vi "TLA_Assembling.vi"(5 "User":string, 6 "stnID":i32, 7 "ProcessIDList":string, 8 "error in (no error)":errorcluster caption="错误输入（无错误）", 9 "JobNo":string, 10 "PCBID":string, 11 "Traceability 引用句柄":refnum<k24>) -> (0 "error out":errorcluster caption="错误输出", 2 ".NET:System.Data.DataTable":T1 {"RemotingFormat" items=["Xml", "Binary"]}, 3 "Traceability 引用句柄输出":refnum<k24>)   [LabVIEW 2014, in "Traceability.lvlib"]
uses:
  D:/webservice/Traceability.dll
  Traceability.dll
  System.Data
  Traceability.lvlib
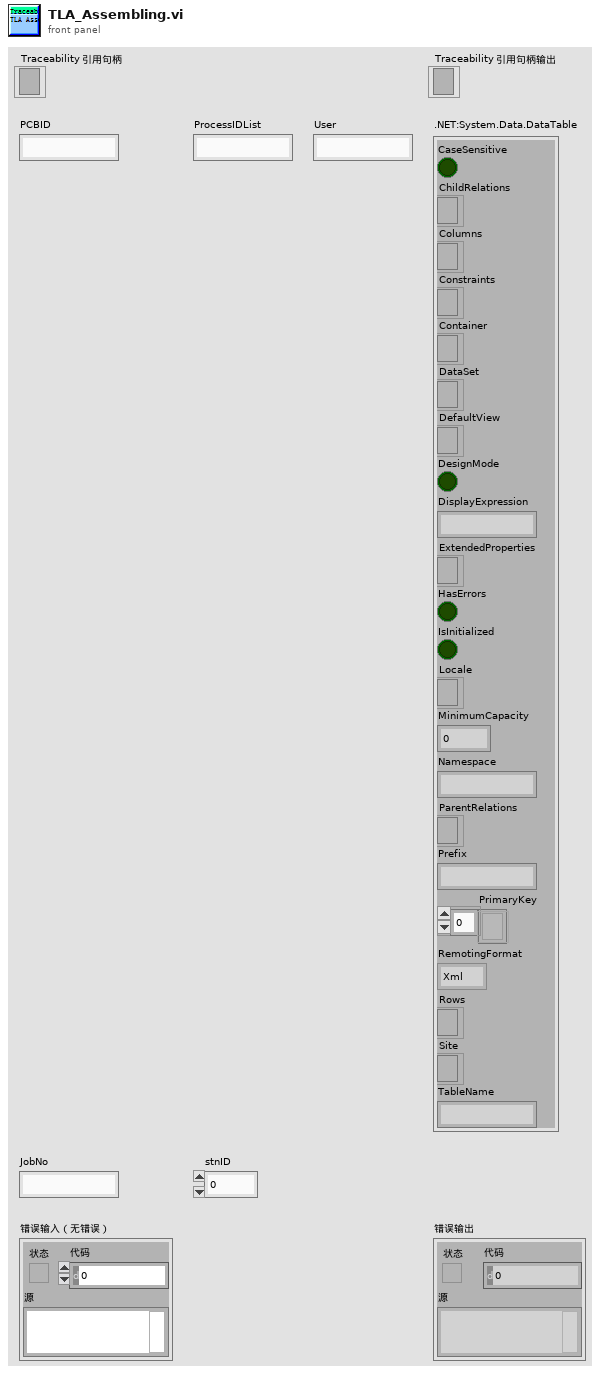
[diagram p1: front panel]
types:
  T1 = cluster{"CaseSensitive":bool, "ChildRelations":refnum<k24>, "Columns":refnum<k24>, "Constraints":refnum<k24>, "Container":refnum<k24>, "DataSet":refnum<k24>, "DefaultView":refnum<k24>, "DesignMode":bool, "DisplayExpression":string, "ExtendedProperties":refnum<k24>, "HasErrors":bool, "IsInitialized":bool, "Locale":refnum<k24>, "MinimumCapacity":i32, "Namespace":string, "ParentRelations":refnum<k24>, "Prefix":string, "PrimaryKey":refnum<k24>[], "RemotingFormat":i32, "Rows":refnum<k24>, "Site":refnum<k24>, "TableName":string}
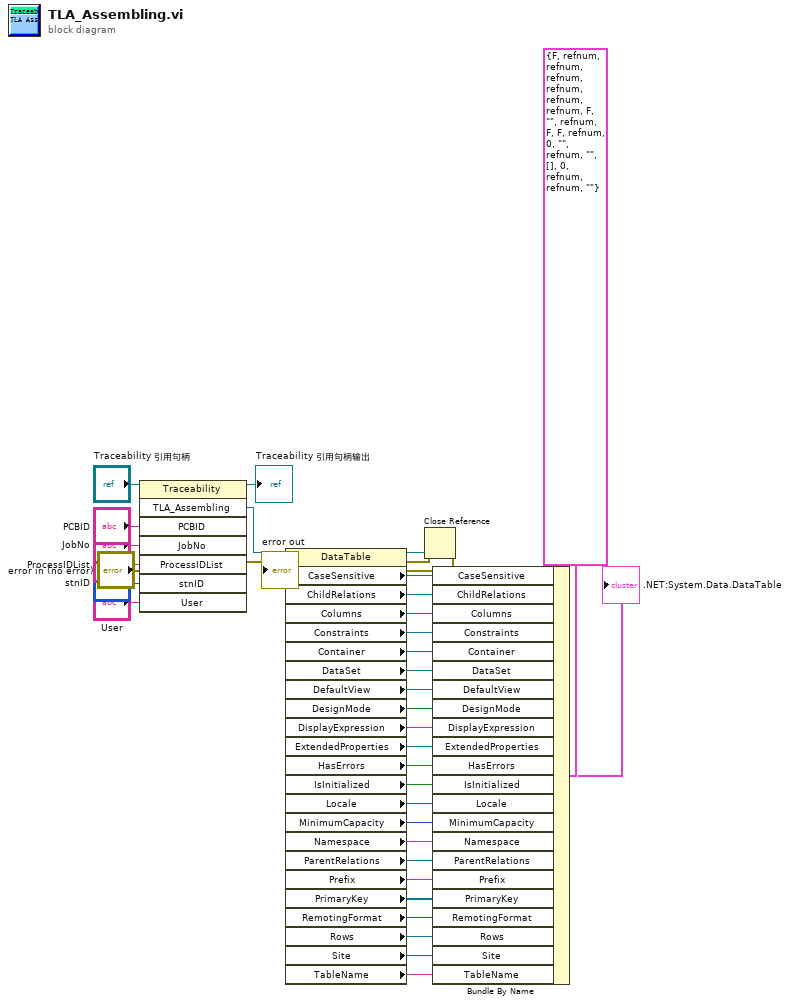
[diagram p0: block diagram]
diagram:
  n1 = invoke class="Traceability" method="TLA_Assembling"(reference="Traceability 引用句柄", error in="error in (no error)", "PCBID"="PCBID", "JobNo"="JobNo", "ProcessIDList"="ProcessIDList", "stnID"="stnID", "User"="User") -> (reference out=→"Traceability 引用句柄输出":refnum<k24>, error out=w4:errorcluster, "TLA_Assembling"=w34:refnum<k24>)  [unwired: 1 in, 5 out]
  n2 = property class="DataTable"(reference=w34, error in=w4) -> (reference out=w3:refnum<k24>, error out=w2:errorcluster, "CaseSensitive"=w31:bool, "ChildRelations"=w30:refnum<k24>, "Columns"=w29:refnum<k24>, "Constraints"=w28:refnum<k24>, "Container"=w27:refnum<k24>, "DataSet"=w26:refnum<k24>, "DefaultView"=w25:refnum<k24>, "DesignMode"=w24:bool, "DisplayExpression"=w23:string, "ExtendedProperties"=w22:refnum<k24>, "HasErrors"=w21:bool, "IsInitialized"=w20:bool, "Locale"=w19:refnum<k24>, "MinimumCapacity"=w18:i32, "Namespace"=w17:string, "ParentRelations"=w16:refnum<k24>, "Prefix"=w15:string, "PrimaryKey"=w14:refnum<k24>[], "RemotingFormat"=w13:i32, "Rows"=w12:refnum<k24>, "Site"=w11:refnum<k24>, "TableName"=w10:string)
  n3 = Close Reference(reference=w3, error in (no error)=w2) -> (error out=→"error out":errorcluster)
  n4 = Bundle By Name(cluster=T1 {"CaseSensitive"=FALSE, "ChildRelations"=refnum, "Columns"=refnum, "Constraints"=refnum, "Container"=refnum, "DataSet"=refnum, "DefaultView"=refnum, "DesignMode"=FALSE, "DisplayExpression"="", "ExtendedProperties"=refnum, "HasErrors"=FALSE, "IsInitialized"=FALSE, "Locale"=refnum, "MinimumCapacity"=0, "Namespace"="", "ParentRelations"=refnum, "Prefix"="", "PrimaryKey"=[], "RemotingFormat"=0, "Rows"=refnum, "Site"=refnum, "TableName"=""} (".NET:System.Data.DataTable"), "CaseSensitive"=w31, "ChildRelations"=w30, "Columns"=w29, "Constraints"=w28, "Container"=w27, "DataSet"=w26, "DefaultView"=w25, "DesignMode"=w24, "DisplayExpression"=w23, "ExtendedProperties"=w22, "HasErrors"=w21, "IsInitialized"=w20, "Locale"=w19, "MinimumCapacity"=w18, "Namespace"=w17, "ParentRelations"=w16, "Prefix"=w15, "PrimaryKey"=w14, "RemotingFormat"=w13, "Rows"=w12, "Site"=w11, "TableName"=w10) -> (→".NET:System.Data.DataTable":T1)
